vi "ClearDMA.vi"(8 "error in (no error)":errorcluster, 11 "FpgaRef5782 In":refnum<class "FpgaRef5782.lvclass">) -> (0 "error out":errorcluster, 3 "FpgaRef5782 Out":refnum<class "FpgaRef5782.lvclass">)   [LabVIEW 2013, in "FpgaRef5782.lvclass"]
uses:
  FpgaRef5782.lvclass
  <vilib>/rvi/interface/nirviMethod/nirviMethod.xnode
  <vilib>/FPGAPlugInAG/Dynamic/niLvFpga_ReadFifo_Dynamic.vi
  <vilib>/rvi/errors/niLvFpgaMergeErrorWithErrorCode.vi
  Scope5782/Config/FPGAref_5782.ctl
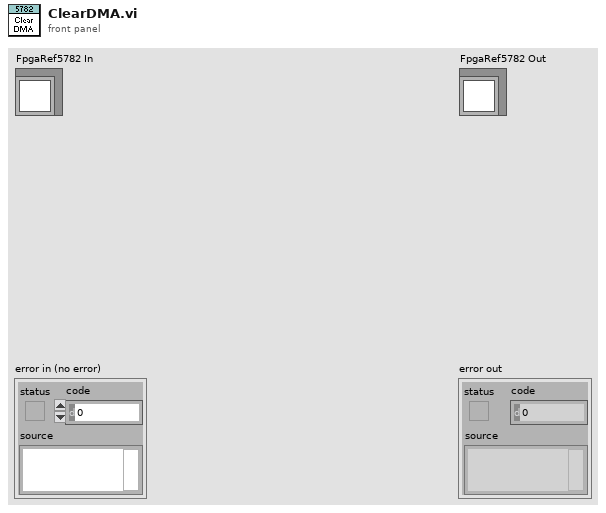
[diagram p1: front panel]
types:
  T1 = typedef "FPGAref_5782.ctl" = refnum<k20>
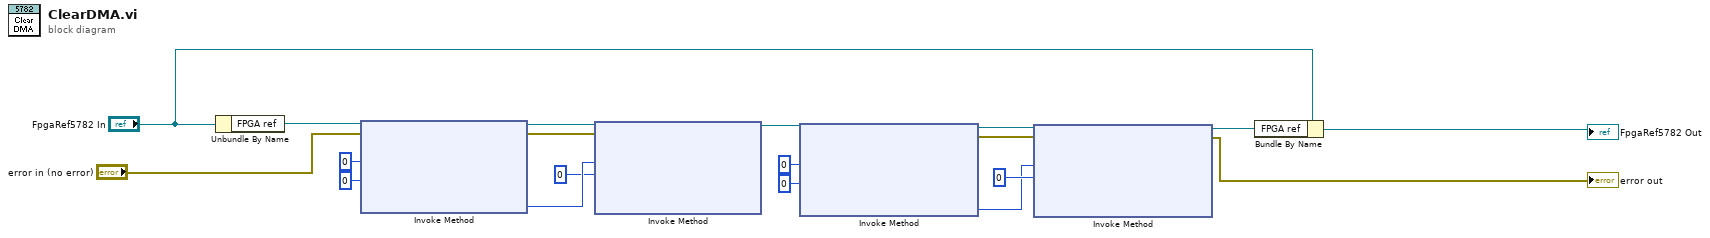
[diagram p0: block diagram]
diagram:
  n1 = Unbundle By Name("FpgaRef5782 In") -> ("FPGA ref"=w6:T1)
  n2 = xnode "Invoke Method"("FPGA VI Reference In"=w6, "error in"="error in (no error)", "Number of Elements"=u32 0, "Timeout (ms)"=0) -> ("FPGA VI Reference Out"=w15:T1, "error out"=w14:errorcluster, "Elements Remaining"=w17:u32)  [unwired: 1 out]
  n3 = xnode "Invoke Method"("FPGA VI Reference In"=w15, "error in"=w14, "Number of Elements"=w17, "Timeout (ms)"=0) -> ("FPGA VI Reference Out"=w7:T1)  [unwired: 3 out]
  n4 = xnode "Invoke Method"("FPGA VI Reference In"=w7, "Number of Elements"=u32 0, "Timeout (ms)"=0) -> ("FPGA VI Reference Out"=w12:T1, "error out"=w13:errorcluster, "Elements Remaining"=w10:u32)  [unwired: 1 in, 1 out]
  n5 = xnode "Invoke Method"("FPGA VI Reference In"=w12, "error in"=w13, "Number of Elements"=w10, "Timeout (ms)"=0) -> ("FPGA VI Reference Out"=w5:T1, "error out"=→"error out":errorcluster)  [unwired: 2 out]
  n6 = Bundle By Name(cluster="FpgaRef5782 In", "FPGA ref"=w5) -> (→"FpgaRef5782 Out":refnum<class "FpgaRef5782.lvclass">)
